vi "Keyence events.vi"(8 "error in":errorcluster, 10 "Variant":variant, 11 "Automation Refnum in":refnum<k7>) -> (0 "error out":errorcluster, 2 "event callback refnum":refnum<k27>)   [LabVIEW 2014]
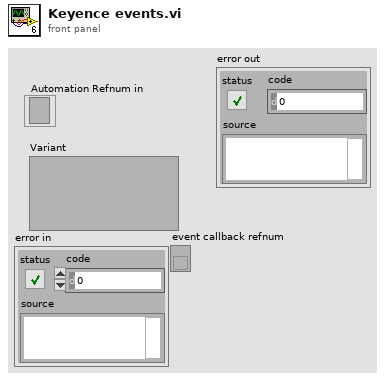
[diagram p1: front panel]
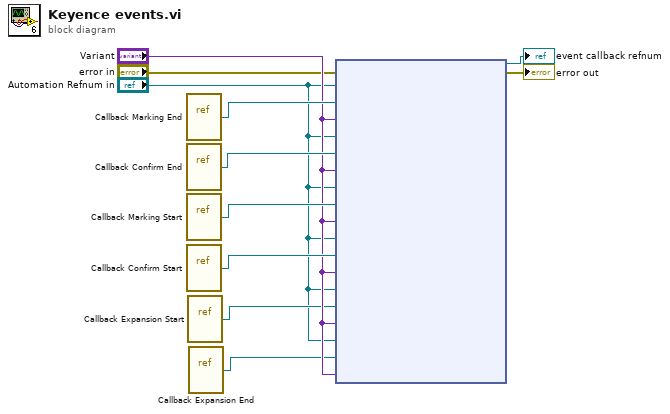
[diagram p0: block diagram]
diagram:
  n1 = vi-ref "Callback Marking End.vi"() -> ("vi reference"=w10:refnum<vi>)
  n2 = vi-ref "Callback Confirm End.vi"() -> ("vi reference"=w11:refnum<vi>)
  n3 = vi-ref "Callback Marking Start.vi"() -> ("vi reference"=w9:refnum<vi>)
  n4 = vi-ref "Callback Confirm Start.vi"() -> ("vi reference"=w8:refnum<vi>)
  n5 = vi-ref "Callback Expansion Start.vi"() -> ("vi reference"=w6:refnum<vi>)
  n6 = vi-ref "Callback Expansion End.vi"() -> ("vi reference"=w5:refnum<vi>)
  n7 = node("error in", "Automation Refnum in", w10, "Variant", "Automation Refnum in", w11, "Variant", "Automation Refnum in", w9, "Variant", "Automation Refnum in", w8, "Variant", "Automation Refnum in", w6, "Variant", "Automation Refnum in", w5, "Variant") -> (→"event callback refnum":refnum<k27>, →"error out":errorcluster)  [unwired: 1 in]
